vi "DataXML closeNode.vi"(8 "error in (no error)":errorcluster, 10 "tag node":refnum<k20>, 11 "DataXML in":refnum<class "DataXML.lvclass">) -> (0 "error out":errorcluster, 3 "DataXML out":refnum<class "DataXML.lvclass">)   [LabVIEW 2018, in "DataXML.lvclass"]
uses:
  DataXML.lvclass
  <vilib>/xml/Close Reference(Node).vi
  <vilib>/xml/NI_XML.lvlib
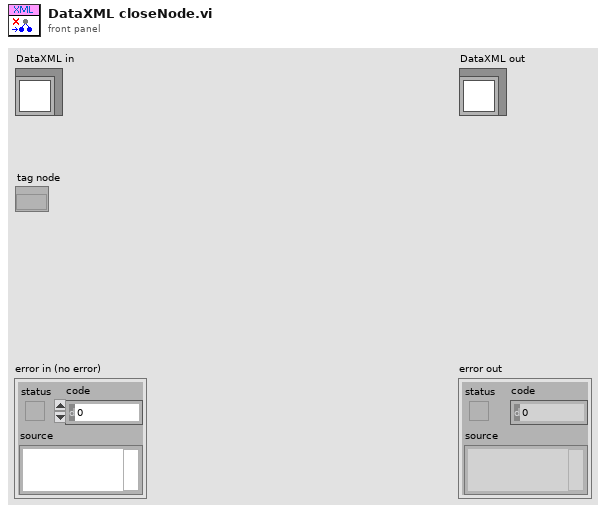
[diagram p1: front panel]
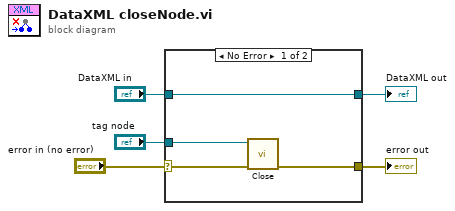
[diagram p0: block diagram]
diagram:
  n1 = case shown="No Error" "error in (no error)" {
    selector: "error in (no error)" -> [w7 w11]
    tunnel: [w6 w11] -> w4
    tunnel: [w9 w10] -> w2
    tunnel: "DataXML in" -> [w9 w10]
    tunnel: "tag node" -> [w8 _]
    frame No Error {
      n2 = call-poly <vilib>:"Close.vi"("error in (no error)"=w7, "node"=w8) -> ("error out"=w6:errorcluster)  [unwired: 7 out]
    }
    frame Error {
    }
  }
  "error out" <- w4
  "DataXML out" <- w2
